vi "RWNoise-Save Data.vi"(0 "RWN Stim":T1, 1 "RW Noise Params":T3, 5 "RW Noise (uV)":dbl, 9 "Spectrum (dB)":waveform(dbl), 11 "error in (no error)":errorcluster, 12 "Expt State":T2) -> (4 "path":path, 14 "Expt State out":T2, 15 "error out":errorcluster)   [LabVIEW 2020]
uses:
  RWNoise Params.ctl
  epl-vi-lib/Utility VIs/Type Defs/Left-Right ring.ctl
  CFTS Main Panel SubVIs/CFTS-Experiment State.ctl
  RWNoise-Stim Params.ctl
  CFTS Main Panel SubVIs/CFTS-Data Type Enum.ctl
  epl-vi-lib/Utility VIs/Math VIs/LinSpace (x0-dx-npts).vi
  epl-vi-lib/Utility VIs/File IO VIs/Configuration File Wrapper VIs/Config-Read Key (string).vi
panel:
  in  "Notes":string
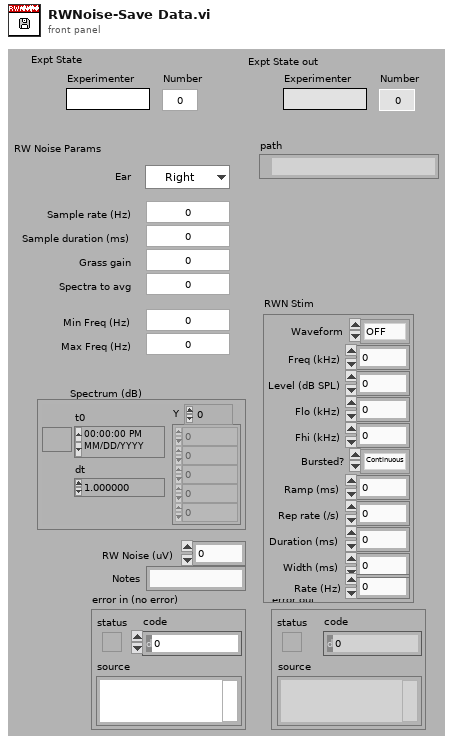
[diagram p1: front panel]
types:
  T1 = typedef "RWNoise-Stim Params.ctl" = cluster{"Waveform":enum16{"OFF", "Tone", "Noise", "Pulses"}, "Freq (kHz)":dbl, "Level (dB SPL)":dbl, "Flo (kHz)":dbl, "Fhi (kHz)":dbl, "Ramp (ms)":dbl, "Rep rate (/s)":dbl, "Bursted?":enum16{"Continuous", "Bursted"}, "Duration (ms)":dbl, "Width (ms)":dbl, "Rate (Hz)":dbl}
  T2 = typedef "CFTS-Experiment State.ctl" = cluster{"Experimenter":string, "Number":u32, "Right":string, "Left":string, "Data Folder":path, "State File":path, "Version Info":string, "End Exposure Time":dbl, "Exposure Duration":string, "Run #":cluster{"CAP":i16, "ABR":i16, "DP":i16, "VsEP":i16, "MeasSeq":i16, "SubSeq":i16, "SFOAE":i16}}
  T3 = typedef "RWNoise Params.ctl" = cluster{"Sample rate (Hz)":dbl, "Sample duration (ms)":dbl, "Grass gain":dbl, "Min Freq (Hz)":dbl, "Max Freq (Hz)":dbl, "Spectra to avg":i32, "Ear":T4}
  T4 = typedef "Left-Right ring.ctl" = enum16{"Right", "Left"}
  T5 = typedef "CFTS-Data Type Enum.ctl" = enum16{"CAP", "ABR", "DP", "VsEP", "MeasSeq", "SFOAE"}
  T6 = enum16{"open", "replace", "create", "open or create", "replace or create", "replace or create with confirmation"}
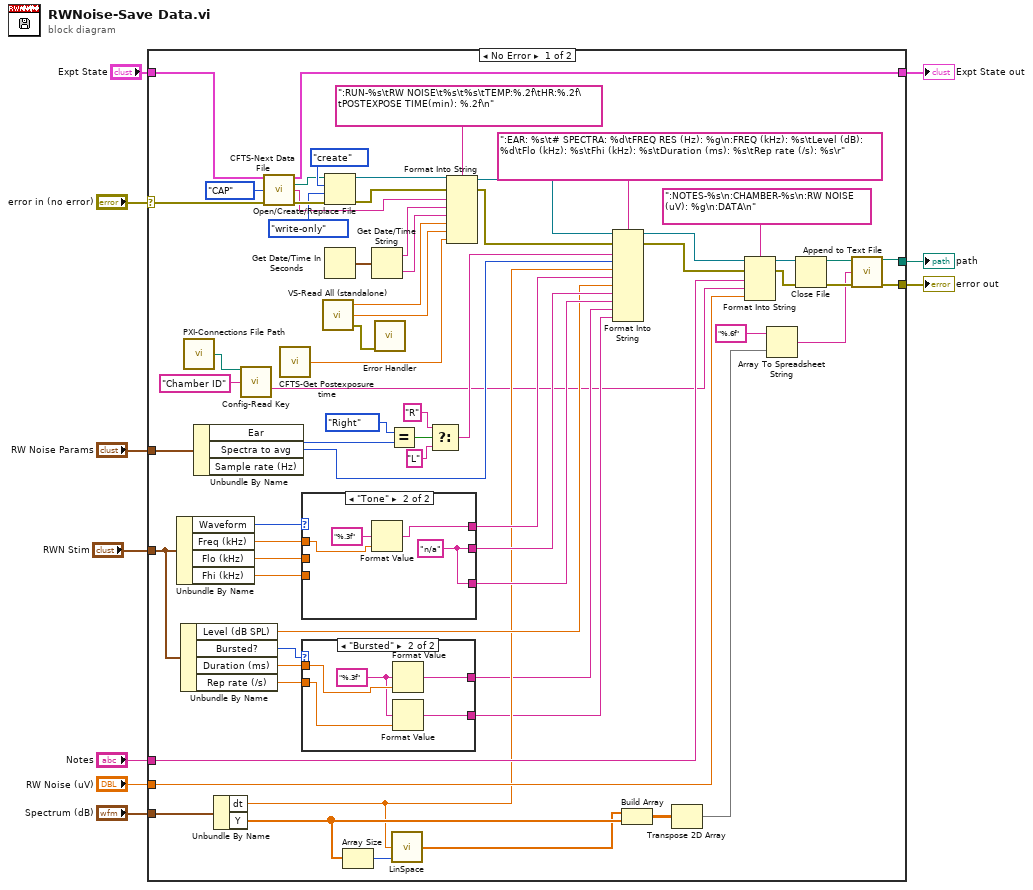
[diagram p0: block diagram]
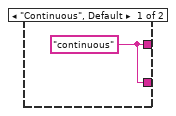
[diagram p2: hidden frame]
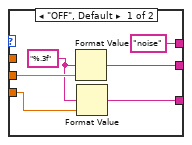
[diagram p3: hidden frame]
diagram:
  n1 = case shown="No Error" "error in (no error)" {
    selector: "error in (no error)" -> [w77 w95]
    tunnel: "RW Noise Params" -> [w65 _]
    tunnel: "Notes" -> [w56 _]
    tunnel: "RW Noise (uV)" -> [w53 _]
    tunnel: [w41 w95] -> w6
    tunnel: [w38 _] -> w5
    tunnel: "Spectrum (dB)" -> [w52 _]
    tunnel: "Expt State" -> [w46 w94]
    tunnel: [w45 w94] -> w2
    tunnel: "RWN Stim" -> [w29 _]
    frame No Error {
      n2 = Unbundle By Name(w29) -> ("Waveform"=w36:enum16{"OFF", "Tone", "Noise", "Pulses"}, "Freq (kHz)"=w35:dbl, "Flo (kHz)"=w33:dbl, "Fhi (kHz)"=w32:dbl)
      n3 = Unbundle By Name(w29) -> ("Level (dB SPL)"=w28:dbl, "Bursted?"=w22:enum16{"Continuous", "Bursted"}, "Duration (ms)"=w21:dbl, "Rep rate (/s)"=w18:dbl)
      n4 = call "PXI-Connections File Path.vi"() -> ("Path"=w12:path)  [unwired: 1 in]
      n5 = Unbundle By Name(w65) -> ("Ear"=w64:T4, "Spectra to avg"=w58:i32)  [unwired: 1 out]
      n6 = Unbundle By Name(w52) -> ("dt"=w25:dbl, "Y"=w26:dbl[])
      n7 = call-poly "Config-Read Key.vi"("configuration file path"=w12, "key"="Chamber ID" ("string")) -> ("value"=w11:string)  [unwired: 10 in, 3 out]
      n8 = call "CFTS-Next Data File.vi"("Expt State"=w46, "Data Type"=CFTS-Data_Type_Enum."CAP", "error in (no error)"=w77) -> ("Expt State out"=w45:T2, "Datafile path"=w48:path, "run #"=w70:string, "error out"=w76:errorcluster)  [unwired: 8 in, 1 out]
      n9 = call "CFTS-Get Postexposure time.vi"() -> ("Postexposure Time (min)"=w49:dbl)  [unwired: 14 in, 1 out]
      n10 = case shown="\"Tone\"" w36 {
        tunnel: w35 -> [_ w92]
        tunnel: ["noise" w91] -> w34
        tunnel: w33 -> [w88 _]
        tunnel: [w87 w90] -> w31
        tunnel: w32 -> [w85 _]
        tunnel: [w84 w90] -> w30
        frame "OFF", Default {
          w86 = "%.3f" ("format string")
          n11 = Format Value(format string=w86, value (0)=w88) -> (output string=w87:string)  [unwired: 1 in]
          n12 = Format Value(format string=w86, value (0)=w85) -> (output string=w84:string)  [unwired: 1 in]
        }
        frame "Tone" {
          w90 = "n/a" ("output string")
          n13 = Format Value(format string="%.3f", value (0)=w92) -> (output string=w91:string)  [unwired: 1 in]
        }
      }
      n14 = case shown="\"Bursted\"" w22 {
        tunnel: w21 -> [_ w83]
        tunnel: [w78 w82] -> w20
        tunnel: w18 -> [_ w81]
        tunnel: [w78 w79] -> w17
        frame "Continuous", Default {
          w78 = "continuous" ("output string")
        }
        frame "Bursted" {
          w80 = "%.3f" ("format string")
          n15 = Format Value(format string=w80, value (0)=w83) -> (output string=w82:string)  [unwired: 1 in]
          n16 = Format Value(format string=w80, value (0)=w81) -> (output string=w79:string)  [unwired: 1 in]
        }
      }
      n17 = call "VS-Read All (standalone).vi"() -> ("error out"=w14:errorcluster, "Heart Rate (bpm)"=w15:dbl, "Temperature (C)"=w16:dbl)  [unwired: 3 in]
      n18 = Open/Create/Replace File(file path (use dialog)=w48, error in=w76, operation (0:open)=T6."create", access (0:read/write)=enum16{"read/write", "read-only", "write-only"}."write-only") -> (refnum out=w73:refnum<file>, error out=w72:errorcluster)  [unwired: 2 in, 1 out]
      n19 = Get Date/Time In Seconds() -> (seconds since 1Jan1904=w69:timestamp)
      n20 = Array Size(array=w26) -> (size(s)=w27:i32)
      n21 = Get Date/Time String(seconds (now)=w69) -> (date string=w51:string, time string=w50:string)  [unwired: 2 in]
      n22 = call "Error Handler.vi"("error in (no error)"=w14) -> ()  [unwired: 13 in, 2 out]
      n23 = Equal?(x=Left-Right_ring."Right" ("y"), y=w64) -> (x = y?=w62:bool)
      n24 = call-poly "LinSpace.vi"("npts"=w27, "dx"=w25) -> ("Array"=w23:dbl[])  [unwired: 2 in, 1 out]
      n25 = Select(t="R", s=w62, f="L") -> (s? t:f=w59:string)
      n26 = Format Into String(format string=":RUN-%s\tRW NOISE\t%s\t%s\tTEMP:%.2f\tHR:%.2f\tPOSTEXPOSE TIME(min): %.2f\n", initial string=w73, error in=w72, w70, w51, w50, w16, w15, w49) -> (resulting string=w67:refnum<file>, error out=w66:errorcluster)
      n27 = Format Into String(format string=":EAR: %s\t# SPECTRA: %d\tFREQ RES (Hz): %g\n:FREQ (kHz): %s\tLevel (dB): %d\tFlo (kHz): %s\tFhi (kHz): %s\tDuration (ms): %s\tRep rate (/s): %s\r", initial string=w67, error in=w66, w59, w58, w25, w34, w28, w31, w30, w20, w17) -> (resulting string=w55:refnum<file>, error out=w54:errorcluster)
      n28 = Build Array(w23, w26) -> (w24:dbl[][])
      n29 = Transpose 2D Array(2D array=w24) -> (transposed array=w19:dbl[][])
      n30 = Format Into String(format string=":NOTES-%s\n:CHAMBER-%s\n:RW NOISE (uV): %g\n:DATA\n", initial string=w55, error in=w54, w56, w11, w53) -> (resulting string=w42:refnum<file>, error out=w43:errorcluster)
      n31 = Array To Spreadsheet String(array=w19, 3:"%.6f" ("format (%.3f)")) -> (spreadsheet string=w37:string)  [unwired: 1 in]
      n32 = Close File(refnum=w42, error in=w43) -> (path=w39:path, error out=w40:errorcluster)
      n33 = call "Append to Text File.vi"("file path"=w39, "text"=w37, "error in (no error)"=w40) -> ("file path out"=w38:path, "error out"=w41:errorcluster)  [unwired: 11 in]
    }
    frame Error {
    }
  }
  "error out" <- w6
  "path" <- w5
  "Expt State out" <- w2
